vi "查看当前子类.vi"(7 "父类":string, 8 "error in (no error)":errorcluster caption="错误输入（无错误）", 10 "Folder Path":path caption="文件夹路径", 11 "查看当前子类 输入":refnum<class "查看当前子类.lvclass">) -> (0 "error out":errorcluster caption="错误输出", 1 "清单名称":string[](array[string]), 2 "数组":refnum<class>[](array[class]), 3 "查看当前子类 输出":refnum<class "查看当前子类.lvclass">)   [LabVIEW 2016, in "查看当前子类.lvclass"]
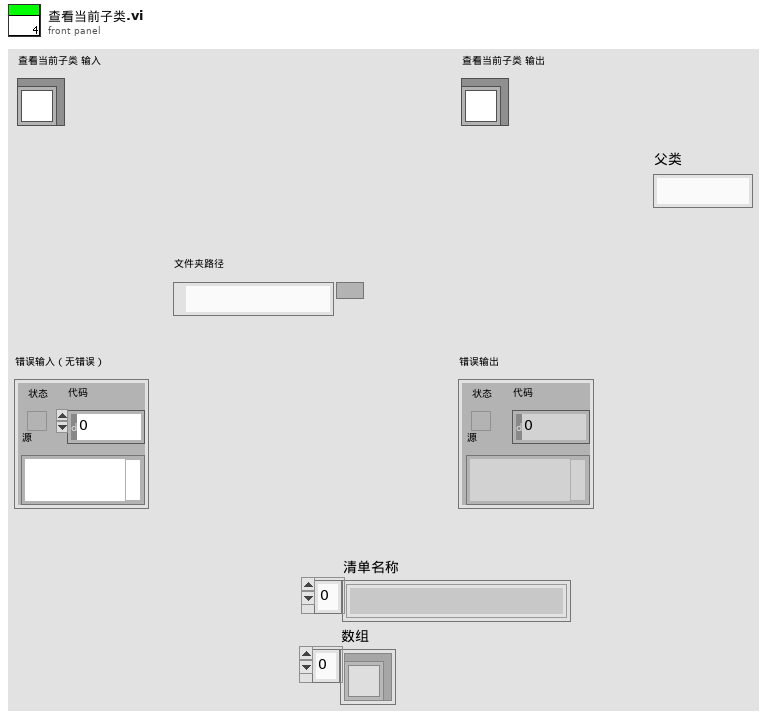
[diagram p1: front panel]
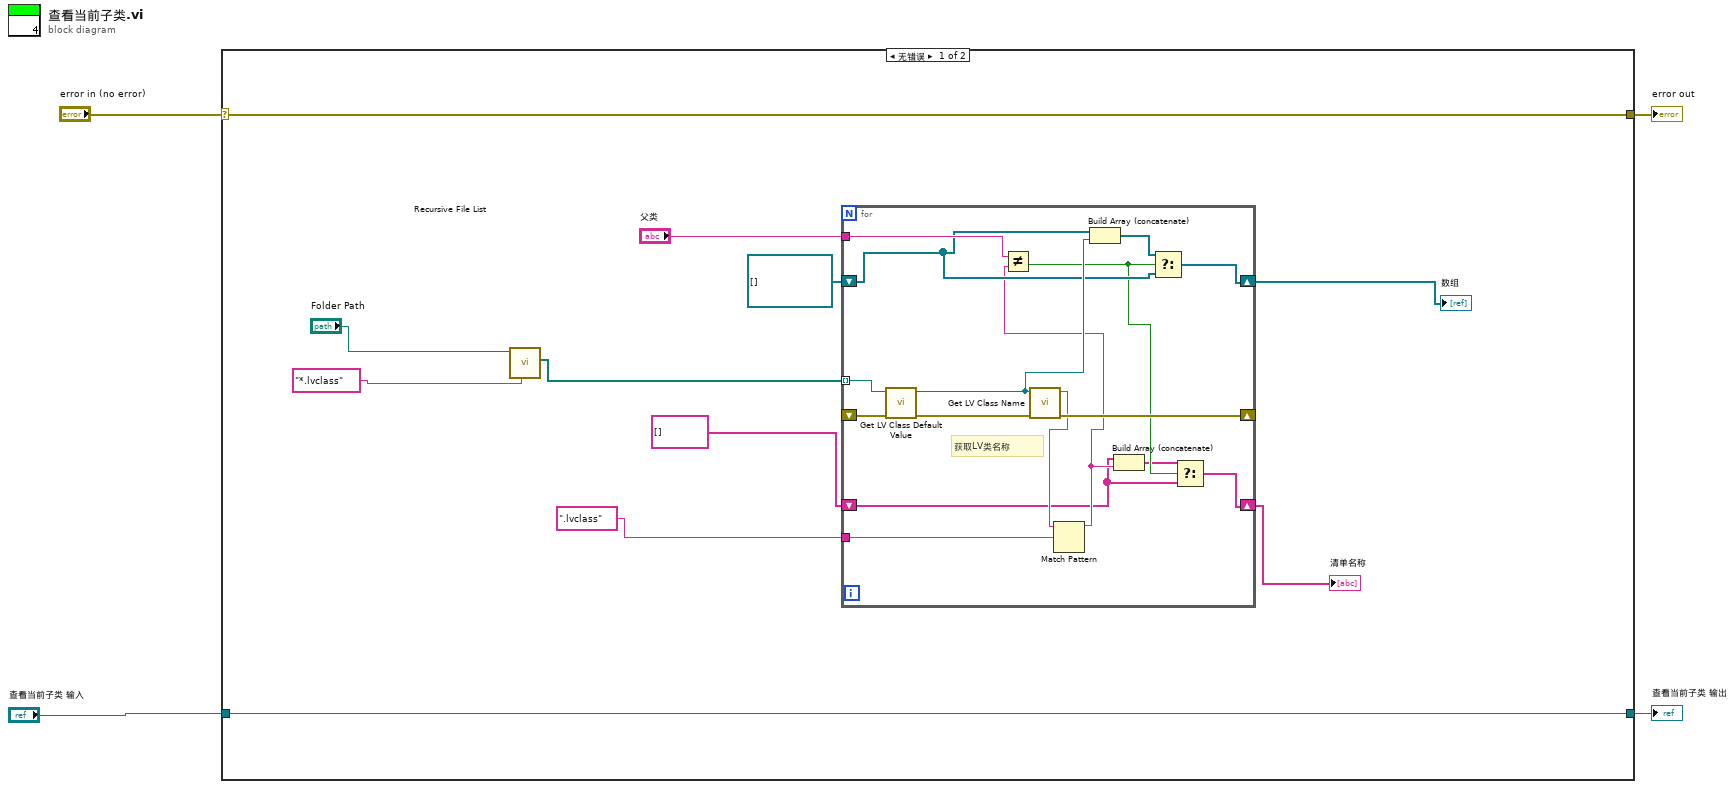
[diagram p0: block diagram]
diagram:
  n1 = case shown="无错误" "error in (no error)" {
    selector: "error in (no error)" -> [w15 w33]
    tunnel: [w15 w33] -> w3
    tunnel: [w12 w32] -> w1
    tunnel: "查看当前子类 输入" -> [w12 w32]
    frame No Error {
      n2 = call <vilib>:"Recursive File List.vi"("pattern"="*.lvclass", "Folder Path"="Folder Path") -> ("All Files in Dir"=w11:path[])  [unwired: 5 in, 4 out]
      n3 = for {
        shift-right: [w29] -> _
        shift-left: _ -> [w31]
        tunnel: w11 -> [w30] mode=indexing
        tunnel: ".lvclass" ("pattern") -> [w26]
        tunnel: "父类" -> [w25]
        shift-right: [w22] -> w8
        shift-left: refnum<class>[] [] -> [w21]
        shift-right: [w17] -> w6
        shift-left: string[] [] -> [w16]
        # "获取LV类名称"
        n4 = call <vilib>:"Get LV Class Default Value.vi"("error in (no error)"=w31, "class path"=w30) -> ("error out"=w28:errorcluster, "object"=w23:refnum<class>)  [unwired: 8 in]
        n5 = call <vilib>:"Get LV Class Name.vi"("error in (no error)"=w28, "object"=w23) -> ("error out"=w29:errorcluster, "class name"=w27:string)  [unwired: 8 in]
        n6 = Match Pattern(string=w27, regular expression=w26) -> (before substring=w19:string)  [unwired: 1 in, 3 out]
        n7 = Not Equal?(x=w25, y=w19) -> (x != y?=w20:bool)
        n8 = Build Array (concatenate)(w21, w23) -> (w24:refnum<class>[])
        n9 = Build Array (concatenate)(w16, w19) -> (w18:string[])
        n10 = Select(t=w24, s=w20, f=w21) -> (s? t:f=w22:refnum<class>[])
        n11 = Select(t=w18, s=w20, f=w16) -> (s? t:f=w17:string[])
      }
      "清单名称" <- w6
      "数组" <- w8
    }
    frame Error {
    }
  }
  "error out" <- w3
  "查看当前子类 输出" <- w1
